vi "Indicate end of heating.vi"(9 "Заданная температура":dbl[](array[numeric]), 11 "Прошлая температура":dbl[](array[numeric])) -> (2 "Нагрев завершен":bool)   [LabVIEW 2016]
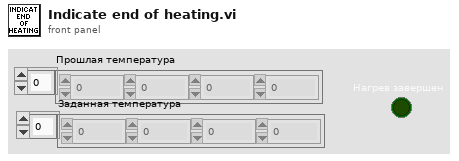
[diagram p1: front panel]
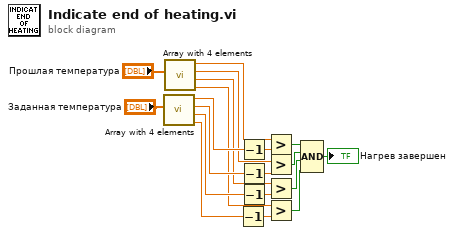
[diagram p0: block diagram]
diagram:
  n1 = call "Array with 4 elements.vi"("Array with 4 elements"="Заданная температура") -> ("element 3"=w6:dbl, "element 2"=w7:dbl, "element 1"=w8:dbl, "element 0"=w9:dbl)  [unwired: 7 in]
  n2 = call "Array with 4 elements.vi"("Array with 4 elements"="Прошлая температура") -> ("element 3"=w1:dbl, "element 2"=w2:dbl, "element 1"=w3:dbl, "element 0"=w4:dbl)  [unwired: 7 in]
  n3 = Decrement(x=w6) -> (x-1=w11:dbl)
  n4 = Decrement(x=w9) -> (x-1=w19:dbl)
  n5 = Decrement(x=w8) -> (x-1=w18:dbl)
  n6 = Decrement(x=w7) -> (x-1=w12:dbl)
  n7 = Greater?(x=w4, y=w19) -> (0:w13:bool)
  n8 = Greater?(x=w3, y=w18) -> (0:w17:bool)
  n9 = Greater?(x=w2, y=w12) -> (0:w16:bool)
  n10 = Greater?(x=w1, y=w11) -> (0:w15:bool)
  n11 = Compound Arithmetic op=AND(w13, w17, w16, w15) -> (→"Нагрев завершен":bool)
